vi "Actor Core.vi"(8 "error in":errorcluster, 11 "Rooms Manager UI in":refnum<class "Rooms Manager UI.lvclass">) -> (0 "error out":errorcluster, 3 "Actor out":refnum<class "Actor.lvclass">)   [LabVIEW 2023, in "Rooms Manager UI.lvlib" / "Rooms Manager UI.lvclass"]
doc: "(<B>Filename</B>: Actor Framework.lvlib:Actor.lvclass:Actor Core.vi)\n\nReceives messages to the actor, reacts to them, and initiates any error handling that may shut the actor down.\n\nDescendant classes may override this VI to append parallel tasks for the actor to complete while it handles messages. Overrides use the Call Parent Class Method node."
uses:
  Rooms Manager UI.lvclass
  C:/Users/bhaghyaraj/Trainings/NI Actor Frameowork/SDLC/UI Base/UI Base/UI Base.lvclass
  C:/Program Files/National Instruments/LabVIEW 2023/vi.lib/ActorFramework/Actor/Actor.lvclass
  <vilib>/ActorFramework/Actor/Actor.lvclass
  Central Data Manager/Central Data Manager/Room Occupancy Status.ctl
  Rooms Manager UI.lvclass/Rooms Manager UI.ctl
  <vilib>/ActorFramework/Actor/Actor.lvclass/Actor.ctl
  <vilib>/ActorFramework/Message Enqueuer/Message Enqueuer.lvclass/Message Enqueuer.ctl
  Rooms Manager UI Messages/Request Room Details Msg/Request Room Details Msg.lvclass/Request Room Details Msg.ctl
  <vilib>/ActorFramework/Message Enqueuer/Init from Existing Queue.vi
  <vilib>/ActorFramework/Message Enqueuer/Enqueue.vi
  <vilib>/ActorFramework/Stop Msg/Stop Msg.lvclass
  C:/Program Files/National Instruments/LabVIEW 2023/vi.lib/ActorFramework/Message/Message.lvclass
  Rooms Manager UI Messages/Request Room Details Msg/Request Room Details Msg.lvclass
  <vilib>/ActorFramework/Message Priority Queue/Priority Enqueue.vi
  <vilib>/ActorFramework/Message Enqueuer/Message Enqueuer.lvclass
  UI Base/UI Base/UI Base.lvclass
  Central Data Manager/Central Data Manager/Central Data Manager.lvclass
panel:
  out "Count":string
  out "Contact Number":string
  out "Guest Name":string
  out "Status":T1
  out "Room Size":string
  out "Room No":string
  out "Rooms Details":T2(array[cluster])
  # "Welcome To Hotel Taj"
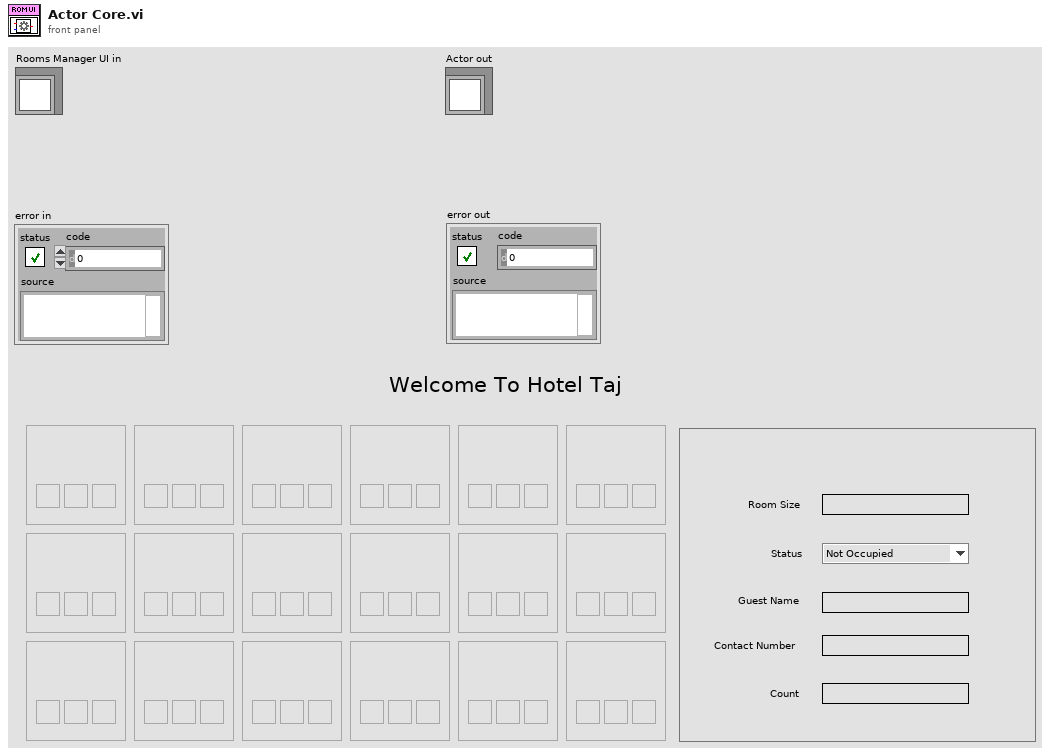
[diagram p1: front panel]
types:
  T1 = typedef "Central Data Manager.lvlib/Central Data Manager.lvclass/Room Occupancy Status.ctl" = enum16{"Not Occupied", "Occupied", "Under Maintainance", "Not Servicable"}
  T2 = cluster{"Room No":string, "Alert":bool, "Occupied":bool, "Maintainance":bool, "IsActive":bool}[][]
  T3 = typedef "LVPoint32TypeDef.ctl" = cluster{"Horizontal":i32, "Vertical":i32}
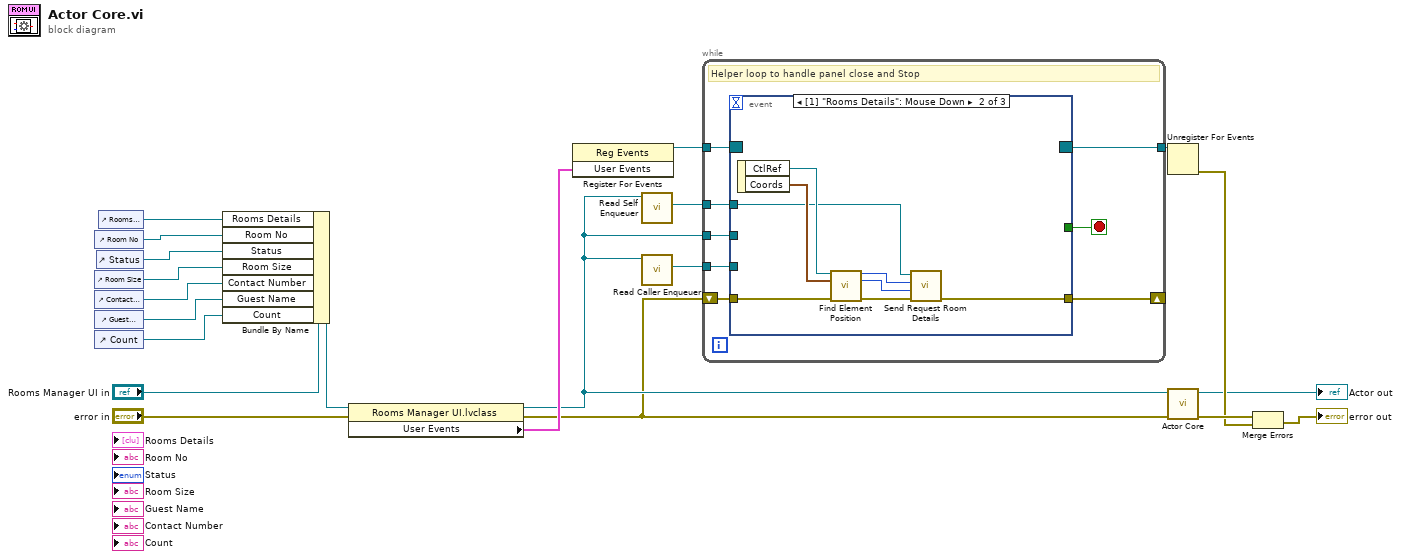
[diagram p0: block diagram]
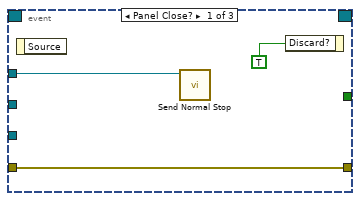
[diagram p2: hidden frame]
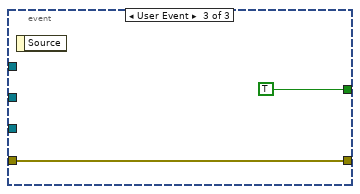
[diagram p3: hidden frame]
diagram:
  n1 = control-ref of="Room No"() -> (w6:refnum<vi>)
  n2 = control-ref of="Room Size"() -> (w4:refnum<vi>)
  n3 = control-ref of="Contact Number"() -> (w1:refnum<vi>)
  n4 = control-ref of="Guest Name"() -> (w2:refnum<vi>)
  n5 = control-ref of="Count"() -> (w3:refnum<vi>)
  n6 = control-ref of="Status"() -> (w5:refnum<vi>)
  n7 = control-ref of="Rooms Details"() -> (w8:refnum<vi>)
  n8 = Bundle By Name(cluster="Rooms Manager UI in", "Rooms Details"=w8, "Room No"=w6, "Status"=w5, "Room Size"=w4, "Contact Number"=w1, "Guest Name"=w2, "Count"=w3) -> (w9:refnum<class "Rooms Manager UI.lvclass">)
  n9 = property class="Rooms Manager UI.lvclass"(reference=w9, error in="error in") -> (reference out=w14:refnum<class "Rooms Manager UI.lvclass">, error out=w7:errorcluster, "User Events"=w17:cluster{"Stop":refnum<user-event>})
  n10 = register-events(w17) -> (reference out=w19:refnum<event-registration>)  [unwired: 2 in, 1 out]
  n11 = call <vilib>:"Read Self Enqueuer.vi"("Actor"=w14) -> ("Self Enqueuer"=w18:refnum<class "Message Enqueuer.lvclass">)  [unwired: 10 in]
  n12 = call <vilib>:"Read Caller Enqueuer.vi"("Actor"=w14) -> ("Caller Enqueuer"=w15:refnum<class "Message Enqueuer.lvclass">)  [unwired: 10 in]
  n13 = while {
    tunnel: w18 -> [w29]
    tunnel: w19 -> [w28]
    tunnel: [w26] -> w20
    tunnel: w15 -> [w25]
    tunnel: w14 -> [w24]
    shift-right: [w22] -> _
    shift-left: w7 -> [w23]
    stop <- w27 stop-if-true
    # "Helper loop to handle panel close and Stop"
    n14 = event shown="[1] \"Rooms Details\": Mouse Down" {
      selector: w28 -> [_ _ _]
      dyn-events: [_ _ _] -> w26
      timeout: _ -> [_ _ _]
      tunnel: w29 -> [w31 w33 _]
      tunnel: [_ _ TRUE] -> w27
      tunnel: w25 -> [_ _ _]
      tunnel: w24 -> [_ _ _]
      tunnel: w23 -> [w30 w38 w41]
      tunnel: [w30 w36 w41] -> w22
      event Panel Close? {
        n15 = event-data() -> ()  [unwired: 1 in, 1 out]
        n16 = call <vilib>:"Send Normal Stop.vi"("Message Enqueuer"=w31) -> ()  [unwired: 10 in, 1 out]
        n17 = event-data("Discard?"=TRUE) -> ()  [unwired: 1 in, 1 out]
      }
      event "Rooms Details": Mouse Down {
        n18 = event-data() -> ("CtlRef"=w40:refnum<vi>, "Coords"=w39:T3)  [unwired: 1 in]
        n19 = call "Find Element Position.vi"("CtlRef"=w40, "Coords"=w39, "error in (no error)"=w38) -> ("Row"=w34:i32, "Column"=w35:i32, "error out"=w37:errorcluster)  [unwired: 10 in]
        n20 = call "Send Request Room Details.vi"("error in (no error)"=w37, "Column"=w35, "Row"=w34, "Message Enqueuer"=w33) -> ("error out"=w36:errorcluster)  [unwired: 6 in, 1 out]
      }
      event User Event {
        n21 = event-data() -> ()  [unwired: 1 in, 1 out]
      }
    }
  }
  n22 = Unregister For Events(event registration refnum=w20) -> (error out=w16:errorcluster)  [unwired: 1 in]
  n23 = call-parent "Actor Core.vi"("error in"=w7, "Actor in"=w14) -> ("error out"=w21:errorcluster, "Actor out"=→"Actor out":refnum<class "Actor.lvclass">)  [unwired: 8 in]
  n24 = Merge Errors(w21, w16) -> (→"error out":errorcluster)
